vi "main_prepare_run.vi"(7 "Runtime":refnum<vi>, 10 "Runtime String":refnum<vi>, 11 "Env. Dir":refnum<vi>) -> ()   [LabVIEW 2019]
uses:
  lib/libSimulationControl/libSimulationControl.lvlib
panel:
  # "*******************************************************************\nBiogas Plant Control\n\nAuthor: Paul Zügel\nGCSC-Frankfurt am Main 2020\n\n*******************************************************************"
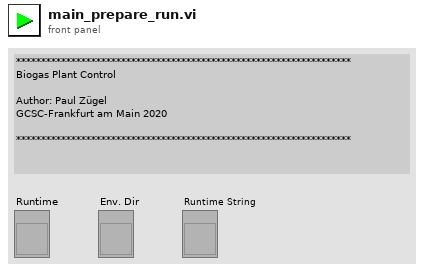
[diagram p1: front panel]
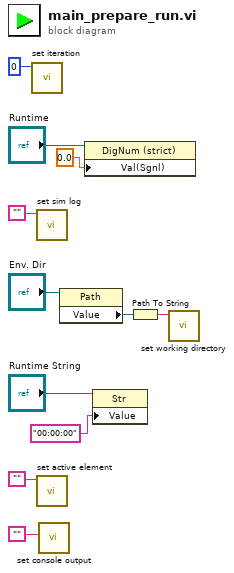
[diagram p0: block diagram]
diagram:
  n1 = call "set iteration.vi"("iter"=0 ("Value")) -> ()  [unwired: 10 in, 1 out]
  n2 = call "set sim log.vi"("log"="") -> ()  [unwired: 10 in, 1 out]
  n3 = call "set active element.vi"("elem"="") -> ()  [unwired: 10 in, 1 out]
  n4 = call "set console output.vi"("console_output"="") -> ()  [unwired: 11 in]
  n5 = property class="Path"(reference="Env. Dir") -> ("Value"=w10:path)  [unwired: 1 in, 2 out]
  n6 = property on="Property Node" class="DigNum (strict)"(reference="Runtime", "Val(Sgnl)"=0.0 ("Value (Signaling)")) -> ()  [unwired: 1 in, 2 out]
  n7 = property on="Property Node" class="Str"(reference="Runtime String", "Value"="00:00:00") -> ()  [unwired: 1 in, 2 out]
  n8 = Path To String(path=w10) -> (string=w11:string)
  n9 = call "set working directory.vi"("dir"=w11) -> ()  [unwired: 10 in, 1 out]
